vi "Noise & Accuracy Processing.vi"(8 "Min Voltage":dbl format="%.2f", 9 "Max Voltage":dbl format="%.2f", 10 "Actual Value":dbl format="%.6f", 11 "Voltage Data":dbl[](array[numeric]) format="%.6f") -> (0 "ENOB (RMS)":dbl format="%.2f", 1 "ENOB (max-min)":dbl format="%.2f", 2 "24-bit Binary Results":T1 {"Error [counts]" format="%.9f"; "max-min" format="%.9f"; "Min" format="%.9f"; "Max" format="%.9f"; "Std Dev (RMS)" format="%.9f"; "Avg" format="%.9f"}, 3 "Results":T2 {"Error [% FS]" format="%.9f"; "Error [volts]" format="%.9f"; "max-min" format="%.9f"; "Min" format="%.9f"; "Max" format="%.9f"; "Std Dev (RMS)" format="%.9f"; "Avg" format="%.9f"}, 4 "Binary Data":dbl[](array[numeric]) format="%.2f", 5 "Results Array":dbl[](array[numeric]) format="%.6f")   [LabVIEW 2024]
uses:
  <vilib>/Analysis/NI_AALBase.lvlib
panel:
  # "Average [volts]"
  # "Std Dev / RMS [volts]"
  # "Max [volts]"
  # "Min [volts]"
  # "Max - Min [volts]"
  # "Error [volts]"
  # "Error [% full span]"
  # "ENOB P-P"
  # "for accuracy calcs"
  # "ENOB RMS"
  # "Average [24-bit counts]"
  # "Std Dev / RMS [counts]"
  # "Max [counts]"
  # "Min [counts]"
  # "Max - Min [counts]"
  # "Error [counts]"
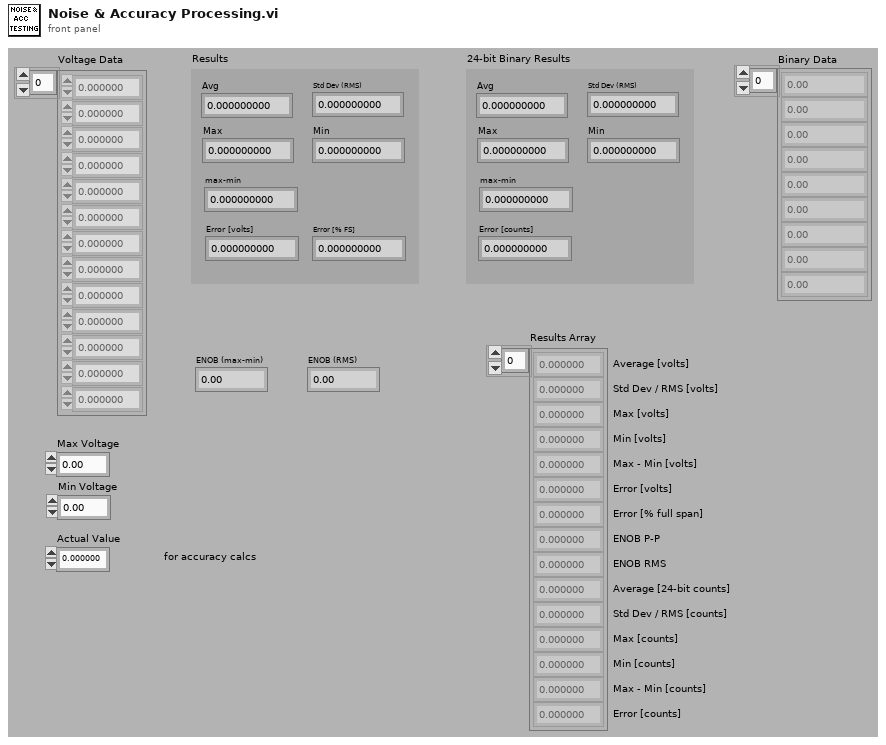
[diagram p1: front panel]
types:
  T1 = cluster{"Avg":dbl, "Std Dev (RMS)":dbl, "Max":dbl, "Min":dbl, "max-min":dbl, "Error [counts]":dbl}
  T2 = cluster{"Avg":dbl, "Std Dev (RMS)":dbl, "Max":dbl, "Min":dbl, "max-min":dbl, "Error [volts]":dbl, "Error [% FS]":dbl}
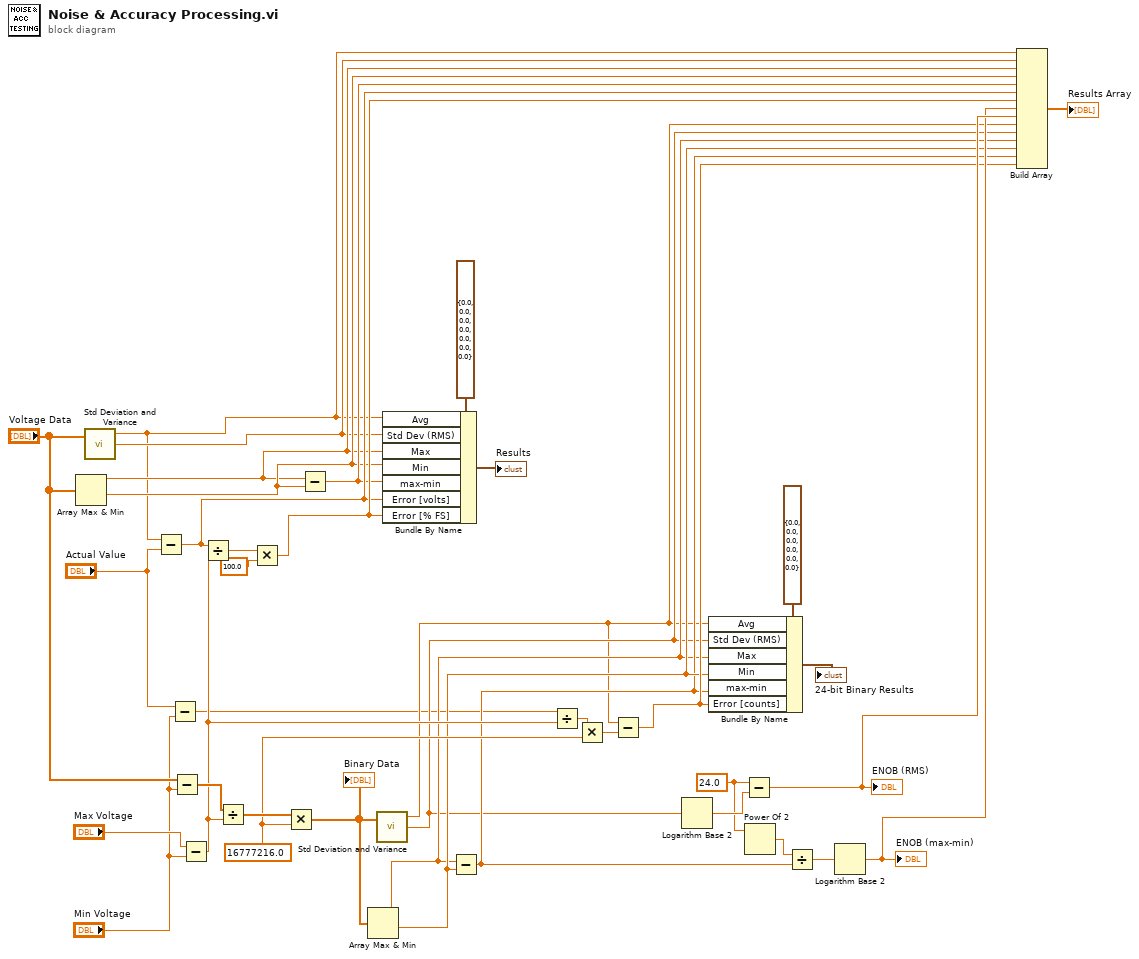
[diagram p0: block diagram]
diagram:
  w20 = 16777216.0 ("x")
  w35 = 24.0 ("x")
  n1 = Array Max & Min(array="Voltage Data") -> (max value=w15:dbl, min value=w16:dbl)  [unwired: 2 out]
  n2 = call <vilib>:"Std Deviation and Variance.vi"("X"="Voltage Data") -> ("mean"=w13:dbl, "standard deviation"=w14:dbl)  [unwired: 1 in, 1 out]
  n3 = Subtract(x=w13, y="Actual Value") -> (x-y=w18:dbl)
  n4 = Subtract(x="Actual Value", y="Min Voltage") -> (x-y=w1:dbl)
  n5 = Subtract(x="Voltage Data", y="Min Voltage") -> (x-y=w31:dbl[])
  n6 = Subtract(x="Max Voltage", y="Min Voltage") -> (x-y=w23:dbl)
  n7 = Divide(x=w18, y=w23) -> (x/y=w27:dbl)
  n8 = Divide(x=w31, y=w23) -> (x/y=w30:dbl[])
  n9 = Multiply(x=w27, y=100.0) -> (x*y=w19:dbl)
  n10 = Multiply(x=w30, y=w20) -> (x*y=w33:dbl[])
  "Binary Data" <- w33
  n11 = Subtract(x=w15, y=w16) -> (x-y=w17:dbl)
  n12 = Array Max & Min(array=w33) -> (max value=w7:dbl, min value=w9:dbl)  [unwired: 2 out]
  n13 = call <vilib>:"Std Deviation and Variance.vi"("X"=w33) -> ("mean"=w5:dbl, "standard deviation"=w6:dbl)  [unwired: 1 in, 1 out]
  n14 = Bundle By Name(cluster=T2 {"Avg"=0.0, "Std Dev (RMS)"=0.0, "Max"=0.0, "Min"=0.0, "max-min"=0.0, "Error [volts]"=0.0, "Error [% FS]"=0.0} ("Results"), "Avg"=w13, "Std Dev (RMS)"=w14, "Max"=w15, "Min"=w16, "max-min"=w17, "Error [volts]"=w18, "Error [% FS]"=w19) -> (→"Results":T2)
  n15 = Subtract(x=w7, y=w9) -> (x-y=w8:dbl)
  n16 = Divide(x=w1, y=w23) -> (x/y=w22:dbl)
  n17 = Multiply(x=w22, y=w20) -> (x*y=w21:dbl)
  n18 = Subtract(x=w5, y=w21) -> (x-y=w10:dbl)
  n19 = Logarithm Base 2(1:w6) -> (0:w36:dbl)
  n20 = Bundle By Name(cluster=T1 {"Avg"=0.0, "Std Dev (RMS)"=0.0, "Max"=0.0, "Min"=0.0, "max-min"=0.0, "Error [counts]"=0.0} ("24-bit Binary Results"), "Avg"=w5, "Std Dev (RMS)"=w6, "Max"=w7, "Min"=w9, "max-min"=w8, "Error [counts]"=w10) -> (→"24-bit Binary Results":T1)
  n21 = Subtract(x=w35, y=w36) -> (x-y=w12:dbl)
  "ENOB (RMS)" <- w12
  n22 = Power Of 2(x=w35) -> (2^x=w37:dbl)
  n23 = Divide(x=w37, y=w8) -> (x/y=w38:dbl)
  n24 = Logarithm Base 2(1:w38) -> (0:w11:dbl)
  "ENOB (max-min)" <- w11
  n25 = Build Array(w13, w14, w15, w16, w17, w18, w19, w11, w12, w5, w6, w7, w9, w8, w10) -> (→"Results Array":dbl[])
